vi "test Data Types.vi"(8 "error in (no error)":errorcluster, 11 "TestCase in":refnum<class "BCD.lvclass">) -> (0 "error out":errorcluster, 3 "TestCase out":refnum<class "BCD.lvclass">)   [LabVIEW 2020, in "BCD.lvclass"]
uses:
  BCD.lvclass
  5f41c702-736d-46cb-8ad7-d7a8da9834e5.vi
  e5a9ed8d-a936-4bcd-9e48-8176d125cb75.vi
  42a7bca9-d213-488f-a610-887b6bb38f81.vi
  d38d9992-20cc-40f4-bca7-551804fb302a.vi
  eb865c1c-101d-43a3-aa66-c96ee64c9e7e.vi
  28633d83-045f-4887-8774-aedc7d445fbd.vi
  0cc24d6e-6748-4204-8650-73a6176edd35.vi
  acbc3292-a6d2-415d-946d-9a3b7456986f.vi
  2d6e40c0-5fb9-4b9b-9465-c2daf76e77d7.vi
  e9447517-9cb6-4615-9498-640261f1ff1f.vi
  4902bbe7-6234-48da-b11f-73dcd207c588.vi
  9cb2f130-739c-4349-ad79-a900f8383a7a.vi
  841edd93-599c-498b-a273-a746ac5e7b71.vi
  6ec24d56-59d0-4064-babc-c34e1fdeb0cb.vi
  3a66866b-dca4-40cf-a6b6-ec7fa99c847f.vi
  da35639a-0b06-4753-9415-a20155f87e80.vi
  28168f98-c96d-478d-8171-4b912791b641.vi
  9cd3ce36-bdf8-4738-a78d-7fe06871668f.vi
  8e77009d-e80f-487d-8924-5583bc157731.vi
  5f41c702-736d-46cb-8ad7-d7a8da9834e5.vi/a54b505c-1216-4ef4-8378-3ceda9d188df.vi
  5f41c702-736d-46cb-8ad7-d7a8da9834e5.vi/136dcdcb-2dd3-4a4d-a796-a8f7a3f8e1ac.vi
  e5a9ed8d-a936-4bcd-9e48-8176d125cb75.vi/0a001d06-2809-4638-8d0b-e017d2157007.vi
  42a7bca9-d213-488f-a610-887b6bb38f81.vi/a54b505c-1216-4ef4-8378-3ceda9d188df.vi
  42a7bca9-d213-488f-a610-887b6bb38f81.vi/136dcdcb-2dd3-4a4d-a796-a8f7a3f8e1ac.vi
  d38d9992-20cc-40f4-bca7-551804fb302a.vi/0a001d06-2809-4638-8d0b-e017d2157007.vi
  eb865c1c-101d-43a3-aa66-c96ee64c9e7e.vi/a54b505c-1216-4ef4-8378-3ceda9d188df.vi
  eb865c1c-101d-43a3-aa66-c96ee64c9e7e.vi/136dcdcb-2dd3-4a4d-a796-a8f7a3f8e1ac.vi
  28633d83-045f-4887-8774-aedc7d445fbd.vi/0a001d06-2809-4638-8d0b-e017d2157007.vi
  0cc24d6e-6748-4204-8650-73a6176edd35.vi/a54b505c-1216-4ef4-8378-3ceda9d188df.vi
  0cc24d6e-6748-4204-8650-73a6176edd35.vi/136dcdcb-2dd3-4a4d-a796-a8f7a3f8e1ac.vi
  acbc3292-a6d2-415d-946d-9a3b7456986f.vi/0a001d06-2809-4638-8d0b-e017d2157007.vi
  2d6e40c0-5fb9-4b9b-9465-c2daf76e77d7.vi/a54b505c-1216-4ef4-8378-3ceda9d188df.vi
  2d6e40c0-5fb9-4b9b-9465-c2daf76e77d7.vi/136dcdcb-2dd3-4a4d-a796-a8f7a3f8e1ac.vi
  e9447517-9cb6-4615-9498-640261f1ff1f.vi/0a001d06-2809-4638-8d0b-e017d2157007.vi
  4902bbe7-6234-48da-b11f-73dcd207c588.vi/a54b505c-1216-4ef4-8378-3ceda9d188df.vi
  4902bbe7-6234-48da-b11f-73dcd207c588.vi/136dcdcb-2dd3-4a4d-a796-a8f7a3f8e1ac.vi
  9cb2f130-739c-4349-ad79-a900f8383a7a.vi/0a001d06-2809-4638-8d0b-e017d2157007.vi
  841edd93-599c-498b-a273-a746ac5e7b71.vi/a54b505c-1216-4ef4-8378-3ceda9d188df.vi
  841edd93-599c-498b-a273-a746ac5e7b71.vi/136dcdcb-2dd3-4a4d-a796-a8f7a3f8e1ac.vi
  6ec24d56-59d0-4064-babc-c34e1fdeb0cb.vi/0a001d06-2809-4638-8d0b-e017d2157007.vi
  3a66866b-dca4-40cf-a6b6-ec7fa99c847f.vi/a54b505c-1216-4ef4-8378-3ceda9d188df.vi
  3a66866b-dca4-40cf-a6b6-ec7fa99c847f.vi/136dcdcb-2dd3-4a4d-a796-a8f7a3f8e1ac.vi
  da35639a-0b06-4753-9415-a20155f87e80.vi/0a001d06-2809-4638-8d0b-e017d2157007.vi
  28168f98-c96d-478d-8171-4b912791b641.vi/a54b505c-1216-4ef4-8378-3ceda9d188df.vi
  28168f98-c96d-478d-8171-4b912791b641.vi/136dcdcb-2dd3-4a4d-a796-a8f7a3f8e1ac.vi
  9cd3ce36-bdf8-4738-a78d-7fe06871668f.vi/0a001d06-2809-4638-8d0b-e017d2157007.vi
  8e77009d-e80f-487d-8924-5583bc157731.vi/a7fcce85-1f75-4572-aeaa-ddfd463a7c5f.vi
  BCD Decode Integer.vi/9a65bfc0-0d77-4ef3-ab58-63df1e1caa90.vi
  5f41c702-736d-46cb-8ad7-d7a8da9834e5.vi/a54b505c-1216-4ef4-8378-3ceda9d188df.vi/a7fcce85-1f75-4572-aeaa-ddfd463a7c5f.vi
  42a7bca9-d213-488f-a610-887b6bb38f81.vi/a54b505c-1216-4ef4-8378-3ceda9d188df.vi/a7fcce85-1f75-4572-aeaa-ddfd463a7c5f.vi
  eb865c1c-101d-43a3-aa66-c96ee64c9e7e.vi/a54b505c-1216-4ef4-8378-3ceda9d188df.vi/a7fcce85-1f75-4572-aeaa-ddfd463a7c5f.vi
  0cc24d6e-6748-4204-8650-73a6176edd35.vi/a54b505c-1216-4ef4-8378-3ceda9d188df.vi/a7fcce85-1f75-4572-aeaa-ddfd463a7c5f.vi
  2d6e40c0-5fb9-4b9b-9465-c2daf76e77d7.vi/a54b505c-1216-4ef4-8378-3ceda9d188df.vi/a7fcce85-1f75-4572-aeaa-ddfd463a7c5f.vi
  4902bbe7-6234-48da-b11f-73dcd207c588.vi/a54b505c-1216-4ef4-8378-3ceda9d188df.vi/a7fcce85-1f75-4572-aeaa-ddfd463a7c5f.vi
  841edd93-599c-498b-a273-a746ac5e7b71.vi/a54b505c-1216-4ef4-8378-3ceda9d188df.vi/a7fcce85-1f75-4572-aeaa-ddfd463a7c5f.vi
  3a66866b-dca4-40cf-a6b6-ec7fa99c847f.vi/a54b505c-1216-4ef4-8378-3ceda9d188df.vi/a7fcce85-1f75-4572-aeaa-ddfd463a7c5f.vi
  28168f98-c96d-478d-8171-4b912791b641.vi/a54b505c-1216-4ef4-8378-3ceda9d188df.vi/a7fcce85-1f75-4572-aeaa-ddfd463a7c5f.vi
  <vilib>/addons/_JKI Toolkits/VI Tester/TestCase.llb/TestCase.lvclass
  Encoding and Decoding.lvlib
  C:/Program Files (x86)/National Instruments/LabVIEW 2020/vi.lib/addons/_JKI Toolkits/VI Tester/TestCase.llb/TestCase.lvclass
panel:
  out "BCD encoded value":bool[](array[boolean])
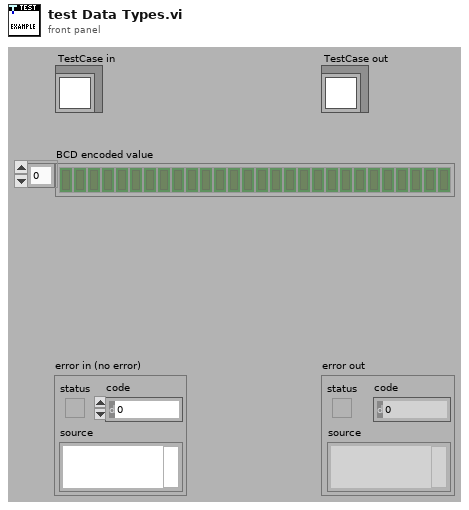
[diagram p1: front panel]
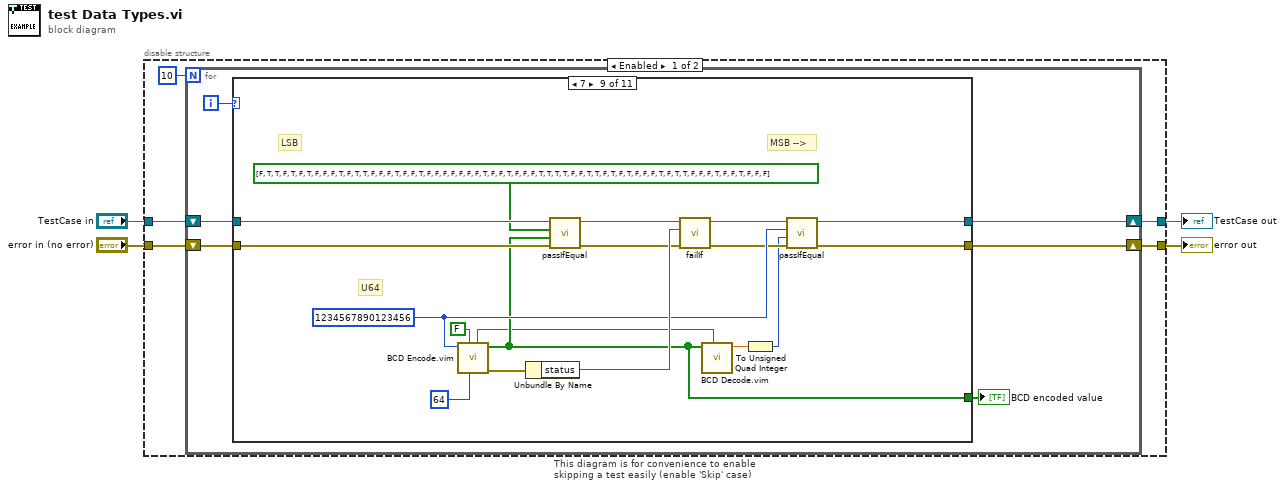
[diagram p0: block diagram]
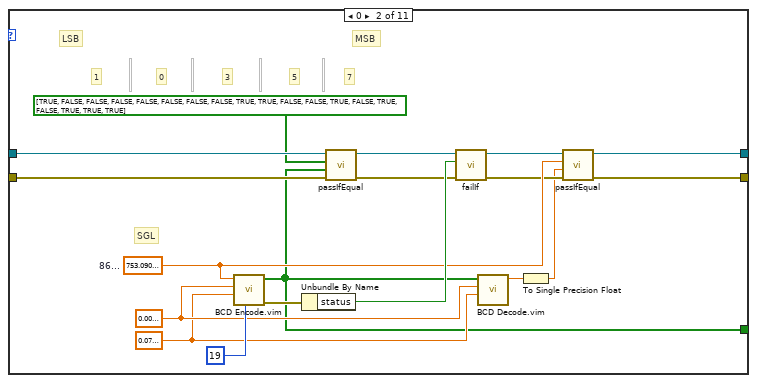
[diagram p3: hidden frame]
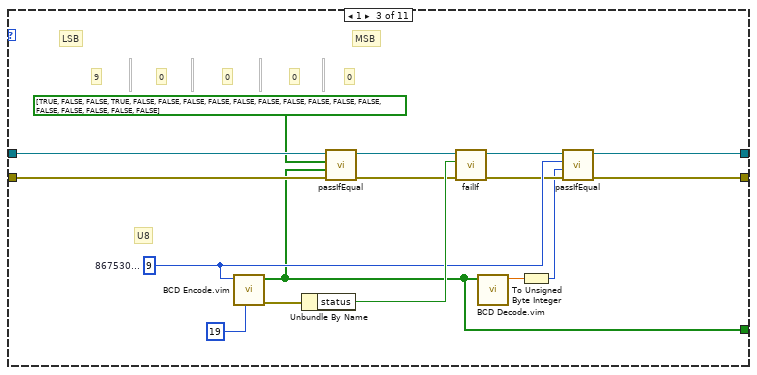
[diagram p4: hidden frame]
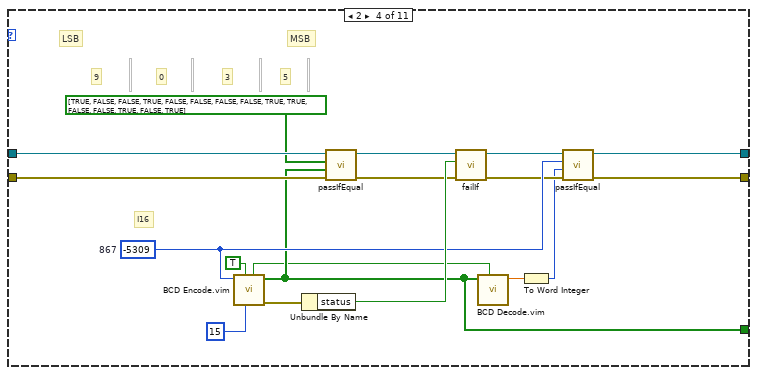
[diagram p5: hidden frame]
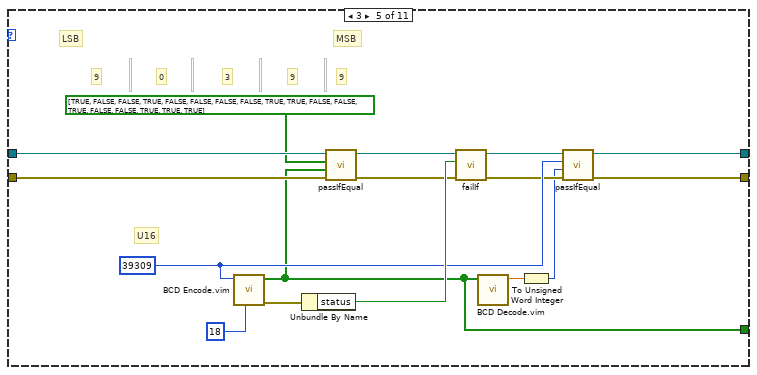
[diagram p6: hidden frame]
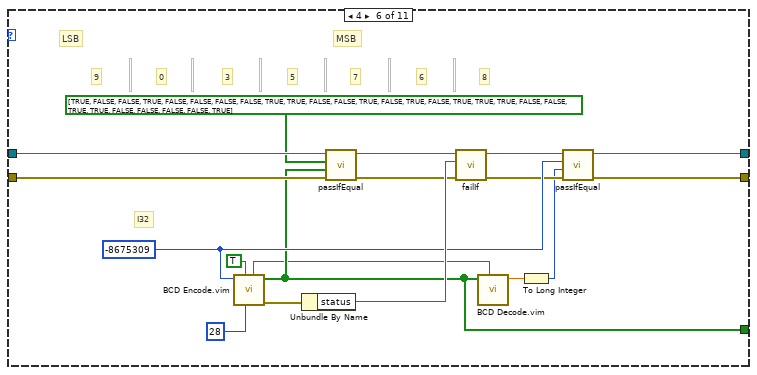
[diagram p7: hidden frame]
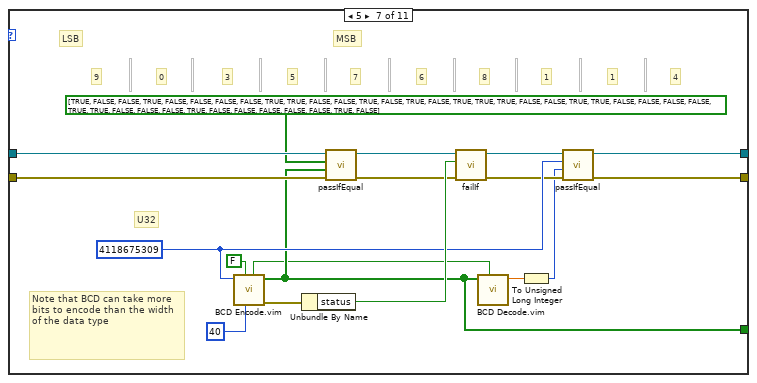
[diagram p8: hidden frame]
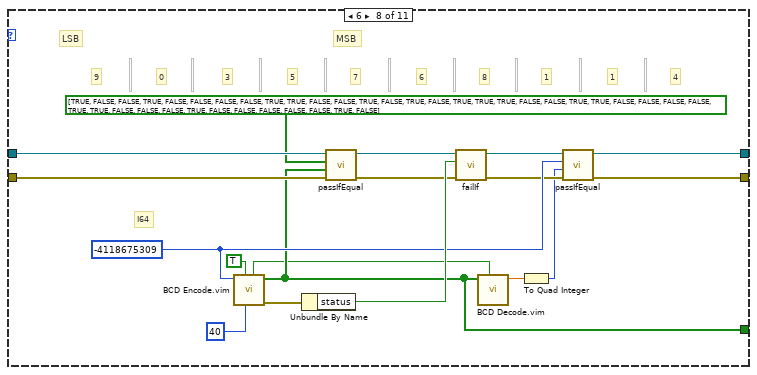
[diagram p9: hidden frame]
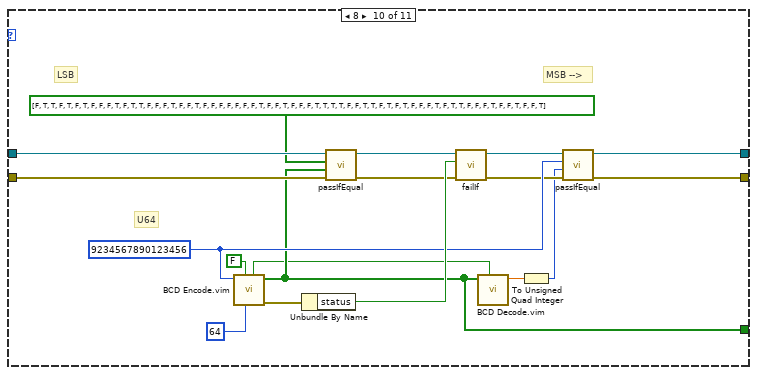
[diagram p10: hidden frame]
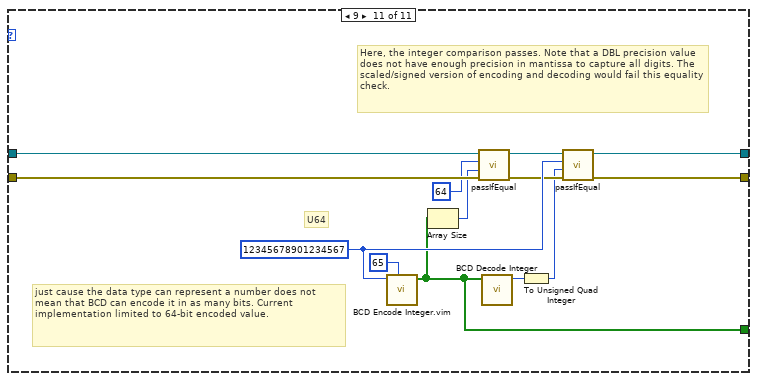
[diagram p11: hidden frame]
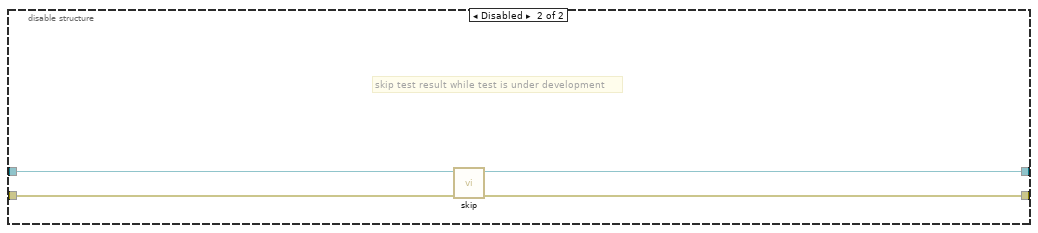
[diagram p12: hidden frame]
diagram:
  n1 = disable-structure "This diagram is for convenience to enable skipping a test easily (enable 'Skip' case)" shown="Enabled" {
    disable-tunnel: "TestCase in" -> [w9 w192]
    disable-tunnel: [w6 w190] -> w1
    disable-tunnel: [w7 w191] -> w3
    disable-tunnel: "error in (no error)" -> [w8 w189]
    frame Enabled {
      n2 = for {
        N: 10 -> [_]
        shift-right: [w12] -> w6
        shift-left: w9 -> [w15]
        shift-right: [w13] -> w7
        shift-left: w8 -> [w14]
        i -> [w11]
        n3 = case shown="7" w11 {
          tunnel: w15 -> [w17 w33 w49 w67 w83 w101 w119 w137 w155 w173 w188]
          tunnel: w14 -> [w16 w32 w48 w66 w82 w100 w118 w136 w154 w172 w187]
          tunnel: [w16 w21 w39 w57 w73 w91 w109 w127 w145 w163 w183] -> w13
          tunnel: [w17 w20 w38 w56 w72 w90 w108 w126 w144 w162 w182] -> w12
          tunnel: [_ w18 w36 w54 w70 w88 w106 w124 w142 w160 w179] -> w10
          frame Default {
          }
          frame 0 {
            w26 = sgl 0.08 ("scale multiplier")
            w27 = sgl 0.01 ("scale multiplier")
            w28 = sgl 753.09  # 86...
            # "SGL"
            # "MSB"
            # "LSB"
            # "1"
            # "0"
            # "3"
            # "5"
            # "7"
            n4 = call "BCD Encode.vim"("data size (bits)"=19, "scale offset"=w26, "scale multiplier"=w27, "value"=w28) -> ("error out"=w30:errorcluster, "BCD encoded value"=w18:bool[])  [unwired: 5 in, 1 out]
            n5 = Unbundle By Name(w30) -> ("status"=w29:bool)
            n6 = call-dynamic "passIfEqual.vi"("error in (no error)"=w32, "y"=w18, "x"=bool[] [TRUE, FALSE, FALSE, FALSE, FALSE, FALSE, FALSE, FALSE, TRUE, TRUE, FALSE, FALSE, TRUE, FALSE, TRUE, FALSE, TRUE, TRUE, TRUE] ("BCD encoded value"), "TestCase in"=w33) -> ("error out"=w24:errorcluster, "TestCase out"=w25:refnum<class "BCD.lvclass">)  [unwired: 6 in]
            n7 = call-dynamic "failIf.vi"("error in (no error)"=w24, "fail"=w29, "TestCase in"=w25) -> ("error out"=w22:errorcluster, "TestCase out"=w23:refnum<class "BCD.lvclass">)  [unwired: 7 in]
            n8 = call "BCD Decode.vim"("scale offset"=w26, "scale multiplier"=w27, "BCD encoded value"=w18) -> ("value"=w34:sgl)  [unwired: 8 in]
            n9 = To Single Precision Float(number=w34) -> (single precision float=w19:sgl)
            n10 = call-dynamic "passIfEqual.vi"("error in (no error)"=w22, "y"=w19, "x"=w28, "TestCase in"=w23) -> ("error out"=w21:errorcluster, "TestCase out"=w20:refnum<class "BCD.lvclass">)  [unwired: 6 in]
          }
          frame 1 {
            w44 = u8 9  # 867530...
            # "U8"
            # "MSB"
            # "LSB"
            # "9"
            # "0"
            # "0"
            # "0"
            # "0"
            n11 = call "BCD Encode.vim"("data size (bits)"=19, "value"=w44) -> ("error out"=w46:errorcluster, "BCD encoded value"=w36:bool[])  [unwired: 7 in, 1 out]
            n12 = Unbundle By Name(w46) -> ("status"=w45:bool)
            n13 = call-dynamic "passIfEqual.vi"("error in (no error)"=w48, "y"=w36, "x"=bool[] [TRUE, FALSE, FALSE, TRUE, FALSE, FALSE, FALSE, FALSE, FALSE, FALSE, FALSE, FALSE, FALSE, FALSE, FALSE, FALSE, FALSE, FALSE, FALSE] ("BCD encoded value"), "TestCase in"=w49) -> ("error out"=w42:errorcluster, "TestCase out"=w43:refnum<class "BCD.lvclass">)  [unwired: 6 in]
            n14 = call-dynamic "failIf.vi"("error in (no error)"=w42, "fail"=w45, "TestCase in"=w43) -> ("error out"=w40:errorcluster, "TestCase out"=w41:refnum<class "BCD.lvclass">)  [unwired: 7 in]
            n15 = call "BCD Decode.vim"("BCD encoded value"=w36) -> ("value"=w50:dbl)  [unwired: 10 in]
            n16 = To Unsigned Byte Integer(number=w50) -> (unsigned 8bit integer=w37:u8)
            n17 = call-dynamic "passIfEqual.vi"("error in (no error)"=w40, "y"=w37, "x"=w44, "TestCase in"=w41) -> ("error out"=w39:errorcluster, "TestCase out"=w38:refnum<class "BCD.lvclass">)  [unwired: 6 in]
          }
          frame 2 {
            w62 = i16 -5309  # 867
            # "I16"
            # "MSB"
            # "LSB"
            # "9"
            # "0"
            # "3"
            # "5"
            n18 = call "BCD Encode.vim"("data size (bits)"=15, "signed"=TRUE, "value"=w62) -> ("error out"=w64:errorcluster, "BCD encoded value"=w54:bool[], "signed?"=w52:bool)  [unwired: 6 in]
            n19 = Unbundle By Name(w64) -> ("status"=w63:bool)
            n20 = call-dynamic "passIfEqual.vi"("error in (no error)"=w66, "y"=w54, "x"=bool[] [TRUE, FALSE, FALSE, TRUE, FALSE, FALSE, FALSE, FALSE, TRUE, TRUE, FALSE, FALSE, TRUE, FALSE, TRUE] ("BCD encoded value"), "TestCase in"=w67) -> ("error out"=w60:errorcluster, "TestCase out"=w61:refnum<class "BCD.lvclass">)  [unwired: 6 in]
            n21 = call-dynamic "failIf.vi"("error in (no error)"=w60, "fail"=w63, "TestCase in"=w61) -> ("error out"=w58:errorcluster, "TestCase out"=w59:refnum<class "BCD.lvclass">)  [unwired: 7 in]
            n22 = call "BCD Decode.vim"("signed"=w52, "BCD encoded value"=w54) -> ("value"=w68:dbl)  [unwired: 9 in]
            n23 = To Word Integer(number=w68) -> (16bit integer=w55:i16)
            n24 = call-dynamic "passIfEqual.vi"("error in (no error)"=w58, "y"=w55, "x"=w62, "TestCase in"=w59) -> ("error out"=w57:errorcluster, "TestCase out"=w56:refnum<class "BCD.lvclass">)  [unwired: 6 in]
          }
          frame 3 {
            w78 = u16 39309 ("867...")
            # "9"
            # "U16"
            # "MSB"
            # "LSB"
            # "9"
            # "0"
            # "3"
            # "9"
            n25 = call "BCD Encode.vim"("data size (bits)"=18, "value"=w78) -> ("error out"=w80:errorcluster, "BCD encoded value"=w70:bool[])  [unwired: 7 in, 1 out]
            n26 = Unbundle By Name(w80) -> ("status"=w79:bool)
            n27 = call-dynamic "passIfEqual.vi"("error in (no error)"=w82, "y"=w70, "x"=bool[] [TRUE, FALSE, FALSE, TRUE, FALSE, FALSE, FALSE, FALSE, TRUE, TRUE, FALSE, FALSE, TRUE, FALSE, FALSE, TRUE, TRUE, TRUE] ("BCD encoded value"), "TestCase in"=w83) -> ("error out"=w76:errorcluster, "TestCase out"=w77:refnum<class "BCD.lvclass">)  [unwired: 6 in]
            n28 = call-dynamic "failIf.vi"("error in (no error)"=w76, "fail"=w79, "TestCase in"=w77) -> ("error out"=w74:errorcluster, "TestCase out"=w75:refnum<class "BCD.lvclass">)  [unwired: 7 in]
            n29 = call "BCD Decode.vim"("BCD encoded value"=w70) -> ("value"=w84:dbl)  [unwired: 10 in]
            n30 = To Unsigned Word Integer(number=w84) -> (unsigned 16bit integer=w71:u16)
            n31 = call-dynamic "passIfEqual.vi"("error in (no error)"=w74, "y"=w71, "x"=w78, "TestCase in"=w75) -> ("error out"=w73:errorcluster, "TestCase out"=w72:refnum<class "BCD.lvclass">)  [unwired: 6 in]
          }
          frame 4 {
            w96 = -8675309 ("867...")
            # "8"
            # "6"
            # "7"
            # "I32"
            # "MSB"
            # "LSB"
            # "9"
            # "0"
            # "3"
            # "5"
            n32 = call "BCD Encode.vim"("data size (bits)"=28, "signed"=TRUE, "value"=w96) -> ("error out"=w98:errorcluster, "BCD encoded value"=w88:bool[], "signed?"=w86:bool)  [unwired: 6 in]
            n33 = Unbundle By Name(w98) -> ("status"=w97:bool)
            n34 = call-dynamic "passIfEqual.vi"("error in (no error)"=w100, "y"=w88, "x"=bool[] [TRUE, FALSE, FALSE, TRUE, FALSE, FALSE, FALSE, FALSE, TRUE, TRUE, FALSE, FALSE, TRUE, FALSE, TRUE, FALSE, TRUE, TRUE, TRUE, FALSE, FALSE, TRUE, TRUE, FALSE, FALSE, FALSE, FALSE, TRUE] ("BCD encoded value"), "TestCase in"=w101) -> ("error out"=w94:errorcluster, "TestCase out"=w95:refnum<class "BCD.lvclass">)  [unwired: 6 in]
            n35 = call-dynamic "failIf.vi"("error in (no error)"=w94, "fail"=w97, "TestCase in"=w95) -> ("error out"=w92:errorcluster, "TestCase out"=w93:refnum<class "BCD.lvclass">)  [unwired: 7 in]
            n36 = call "BCD Decode.vim"("signed"=w86, "BCD encoded value"=w88) -> ("value"=w102:dbl)  [unwired: 9 in]
            n37 = To Long Integer(number=w102) -> (32bit integer=w89:i32)
            n38 = call-dynamic "passIfEqual.vi"("error in (no error)"=w92, "y"=w89, "x"=w96, "TestCase in"=w93) -> ("error out"=w91:errorcluster, "TestCase out"=w90:refnum<class "BCD.lvclass">)  [unwired: 6 in]
          }
          frame 5 {
            w114 = u32 4118675309 ("867...")
            # "Note that BCD can take more bits to encode than the width of the data type"
            # "4"
            # "1"
            # "1"
            # "8"
            # "6"
            # "7"
            # "U32"
            # "MSB"
            # "LSB"
            # "9"
            # "0"
            # "3"
            # "5"
            n39 = call "BCD Encode.vim"("data size (bits)"=40, "signed"=FALSE, "value"=w114) -> ("error out"=w116:errorcluster, "BCD encoded value"=w106:bool[], "signed?"=w104:bool)  [unwired: 6 in]
            n40 = Unbundle By Name(w116) -> ("status"=w115:bool)
            n41 = call-dynamic "passIfEqual.vi"("error in (no error)"=w118, "y"=w106, "x"=bool[] [TRUE, FALSE, FALSE, TRUE, FALSE, FALSE, FALSE, FALSE, TRUE, TRUE, FALSE, FALSE, TRUE, FALSE, TRUE, FALSE, TRUE, TRUE, TRUE, FALSE, FALSE, TRUE, TRUE, FALSE, FALSE, FALSE, FALSE, TRUE, TRUE, FALSE, FALSE, FALSE, TRUE, FALSE, FALSE, FALSE, FALSE, FALSE, TRUE, FALSE] ("BCD encoded value"), "TestCase in"=w119) -> ("error out"=w112:errorcluster, "TestCase out"=w113:refnum<class "BCD.lvclass">)  [unwired: 6 in]
            n42 = call-dynamic "failIf.vi"("error in (no error)"=w112, "fail"=w115, "TestCase in"=w113) -> ("error out"=w110:errorcluster, "TestCase out"=w111:refnum<class "BCD.lvclass">)  [unwired: 7 in]
            n43 = call "BCD Decode.vim"("signed"=w104, "BCD encoded value"=w106) -> ("value"=w120:dbl)  [unwired: 9 in]
            n44 = To Unsigned Long Integer(number=w120) -> (unsigned 32bit integer=w107:u32)
            n45 = call-dynamic "passIfEqual.vi"("error in (no error)"=w110, "y"=w107, "x"=w114, "TestCase in"=w111) -> ("error out"=w109:errorcluster, "TestCase out"=w108:refnum<class "BCD.lvclass">)  [unwired: 6 in]
          }
          frame 6 {
            w132 = i64 -4118675309 ("867...")
            # "4"
            # "1"
            # "1"
            # "8"
            # "6"
            # "7"
            # "I64"
            # "MSB"
            # "LSB"
            # "9"
            # "0"
            # "3"
            # "5"
            n46 = call "BCD Encode.vim"("data size (bits)"=40, "signed"=TRUE, "value"=w132) -> ("error out"=w134:errorcluster, "BCD encoded value"=w124:bool[], "signed?"=w122:bool)  [unwired: 6 in]
            n47 = Unbundle By Name(w134) -> ("status"=w133:bool)
            n48 = call-dynamic "passIfEqual.vi"("error in (no error)"=w136, "y"=w124, "x"=bool[] [TRUE, FALSE, FALSE, TRUE, FALSE, FALSE, FALSE, FALSE, TRUE, TRUE, FALSE, FALSE, TRUE, FALSE, TRUE, FALSE, TRUE, TRUE, TRUE, FALSE, FALSE, TRUE, TRUE, FALSE, FALSE, FALSE, FALSE, TRUE, TRUE, FALSE, FALSE, FALSE, TRUE, FALSE, FALSE, FALSE, FALSE, FALSE, TRUE, FALSE] ("BCD encoded value"), "TestCase in"=w137) -> ("error out"=w130:errorcluster, "TestCase out"=w131:refnum<class "BCD.lvclass">)  [unwired: 6 in]
            n49 = call-dynamic "failIf.vi"("error in (no error)"=w130, "fail"=w133, "TestCase in"=w131) -> ("error out"=w128:errorcluster, "TestCase out"=w129:refnum<class "BCD.lvclass">)  [unwired: 7 in]
            n50 = call "BCD Decode.vim"("signed"=w122, "BCD encoded value"=w124) -> ("value"=w138:dbl)  [unwired: 9 in]
            n51 = To Quad Integer(1:w138) -> (0:w125:i64)
            n52 = call-dynamic "passIfEqual.vi"("error in (no error)"=w128, "y"=w125, "x"=w132, "TestCase in"=w129) -> ("error out"=w127:errorcluster, "TestCase out"=w126:refnum<class "BCD.lvclass">)  [unwired: 6 in]
          }
          frame 7 {
            w150 = u64 1234567890123456 ("867...")
            # "U64"
            # "MSB -->"
            # "LSB"
            n53 = call "BCD Encode.vim"("data size (bits)"=64, "signed"=FALSE, "value"=w150) -> ("error out"=w152:errorcluster, "BCD encoded value"=w142:bool[], "signed?"=w140:bool)  [unwired: 6 in]
            n54 = Unbundle By Name(w152) -> ("status"=w151:bool)
            n55 = call-dynamic "passIfEqual.vi"("error in (no error)"=w154, "y"=w142, "x"=bool[] [FALSE, TRUE, TRUE, FALSE, TRUE, FALSE, TRUE, FALSE, FALSE, FALSE, TRUE, FALSE, TRUE, TRUE, FALSE, FALSE, FALSE, TRUE, FALSE, FALSE, TRUE, FALSE, FALSE, FALSE, FALSE, FALSE, FALSE, FALSE, TRUE, FALSE, FALSE, TRUE, FALSE, FALSE, FALSE, TRUE, TRUE, TRUE, TRUE, FALSE, FALSE, TRUE, TRUE, FALSE, TRUE, FALSE, TRUE, FALSE, FALSE, FALSE, TRUE, FALSE, TRUE, TRUE, FALSE, FALSE, FALSE, TRUE, FALSE, FALSE, TRUE, FALSE, FALSE, FALSE] ("BCD encoded value"), "TestCase in"=w155) -> ("error out"=w148:errorcluster, "TestCase out"=w149:refnum<class "BCD.lvclass">)  [unwired: 6 in]
            n56 = call-dynamic "failIf.vi"("error in (no error)"=w148, "fail"=w151, "TestCase in"=w149) -> ("error out"=w146:errorcluster, "TestCase out"=w147:refnum<class "BCD.lvclass">)  [unwired: 7 in]
            n57 = call "BCD Decode.vim"("signed"=w140, "BCD encoded value"=w142) -> ("value"=w156:dbl)  [unwired: 9 in]
            n58 = To Unsigned Quad Integer(1:w156) -> (0:w143:u64)
            n59 = call-dynamic "passIfEqual.vi"("error in (no error)"=w146, "y"=w143, "x"=w150, "TestCase in"=w147) -> ("error out"=w145:errorcluster, "TestCase out"=w144:refnum<class "BCD.lvclass">)  [unwired: 6 in]
          }
          frame 8 {
            w168 = u64 9234567890123456 ("867...")
            # "U64"
            # "MSB -->"
            # "LSB"
            n60 = call "BCD Encode.vim"("data size (bits)"=64, "signed"=FALSE, "value"=w168) -> ("error out"=w170:errorcluster, "BCD encoded value"=w160:bool[], "signed?"=w158:bool)  [unwired: 6 in]
            n61 = Unbundle By Name(w170) -> ("status"=w169:bool)
            n62 = call-dynamic "passIfEqual.vi"("error in (no error)"=w172, "y"=w160, "x"=bool[] [FALSE, TRUE, TRUE, FALSE, TRUE, FALSE, TRUE, FALSE, FALSE, FALSE, TRUE, FALSE, TRUE, TRUE, FALSE, FALSE, FALSE, TRUE, FALSE, FALSE, TRUE, FALSE, FALSE, FALSE, FALSE, FALSE, FALSE, FALSE, TRUE, FALSE, FALSE, TRUE, FALSE, FALSE, FALSE, TRUE, TRUE, TRUE, TRUE, FALSE, FALSE, TRUE, TRUE, FALSE, TRUE, FALSE, TRUE, FALSE, FALSE, FALSE, TRUE, FALSE, TRUE, TRUE, FALSE, FALSE, FALSE, TRUE, FALSE, FALSE, TRUE, FALSE, FALSE, TRUE] ("BCD encoded value"), "TestCase in"=w173) -> ("error out"=w166:errorcluster, "TestCase out"=w167:refnum<class "BCD.lvclass">)  [unwired: 6 in]
            n63 = call-dynamic "failIf.vi"("error in (no error)"=w166, "fail"=w169, "TestCase in"=w167) -> ("error out"=w164:errorcluster, "TestCase out"=w165:refnum<class "BCD.lvclass">)  [unwired: 7 in]
            n64 = call "BCD Decode.vim"("signed"=w158, "BCD encoded value"=w160) -> ("value"=w174:dbl)  [unwired: 9 in]
            n65 = To Unsigned Quad Integer(1:w174) -> (0:w161:u64)
            n66 = call-dynamic "passIfEqual.vi"("error in (no error)"=w164, "y"=w161, "x"=w168, "TestCase in"=w165) -> ("error out"=w163:errorcluster, "TestCase out"=w162:refnum<class "BCD.lvclass">)  [unwired: 6 in]
          }
          frame 9 {
            w186 = u64 12345678901234567 ("867...")
            # "Here, the integer comparison passes. Note that a DBL precision value does not have enough precision in mantissa to capture all digits. The scaled/signed version of encoding and decoding would fail this equality check."
            # "just cause the data type can represent a number does not mean that BCD can encode it in as many bits. Current implementation limited to 64-bit encoded value."
            # "U64"
            n67 = call "BCD Encode Integer.vim"("data size (bits)"=65, "integer"=w186) -> ("BCD encoded value"=w179:bool[])  [unwired: 8 in, 1 out]
            n68 = Array Size(array=w179) -> (size(s)=w178:i32)
            n69 = call-dynamic "passIfEqual.vi"("error in (no error)"=w187, "y"=w178, "x"=64 ("size(s)"), "TestCase in"=w188) -> ("error out"=w184:errorcluster, "TestCase out"=w185:refnum<class "BCD.lvclass">)  [unwired: 6 in]
            n70 = call "BCD Decode Integer.vi"("BCD encoded value"=w179) -> ("integer"=w180:i64)  [unwired: 10 in]
            n71 = To Unsigned Quad Integer(1:w180) -> (0:w181:u64)
            n72 = call-dynamic "passIfEqual.vi"("error in (no error)"=w184, "y"=w181, "x"=w186, "TestCase in"=w185) -> ("error out"=w183:errorcluster, "TestCase out"=w182:refnum<class "BCD.lvclass">)  [unwired: 6 in]
          }
        }
        "BCD encoded value" <- w10
      }
    }
    frame Disabled {
      # "skip test result while test is under development"
      n73 = call <vilib>:"skip.vi"("error in (no error)"=w189, "TestCase in"=w192) -> ("error out"=w191:errorcluster, "TestCase out"=w190:refnum<class "BCD.lvclass">)  [unwired: 8 in]
    }
  }
  "error out" <- w3
  "TestCase out" <- w1
